vi "Overlay Feature Points-Sized.vi"(6 "Color":u32(colorbox)=16711680, 7 "Group":string, 8 "error in":errorcluster, 9 "Size":i32=5, 10 "Feature Points":cluster{"X":sgl, "Y":sgl}[](array[cluster]), 11 "Image":T1) -> (0 "error out":errorcluster, 3 "Image Out":T1)   [LabVIEW 2018]
doc: "Overlay targets at the location of the feature points in the specified colors."
uses:
  <vilib>/vision/Image Controls.llb/IMAQ Image.ctl
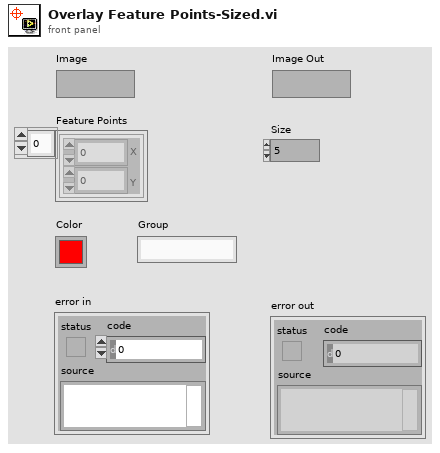
[diagram p1: front panel]
types:
  T1 = typedef "IMAQ Image.ctl" = refnum<image>
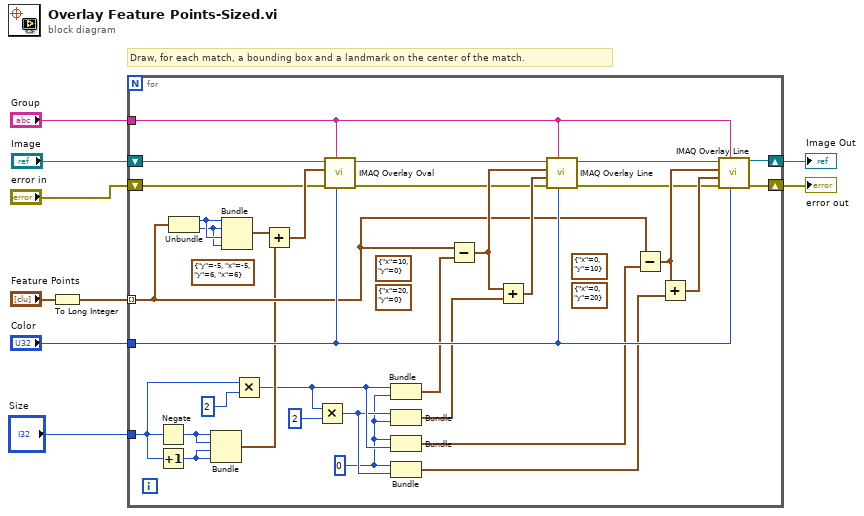
[diagram p0: block diagram]
diagram:
  # "Draw, for each match, a bounding box and a landmark on the center of the match."
  n1 = To Long Integer(number="Feature Points") -> (32bit integer=w6:cluster{"X":i32, "Y":i32}[])
  n2 = for {
    shift-right: [w39] -> w8
    shift-left: "Image" -> [w41]
    tunnel: w6 -> [w23] mode=indexing
    tunnel: "Color" -> [w40]
    tunnel: "Group" -> [w24]
    shift-right: [w25] -> w2
    shift-left: "error in" -> [w28]
    tunnel: "Size" -> [w19]
    w12 = 0 ("y")
    (unwired) cluster{"y":i32, "x":i32, "y":i32, "x":i32} {"y"=-5, "x"=-5, "y"=6, "x"=6} ("y")
    (unwired) cluster{"x":i32, "y":i32} {"x"=0, "y"=20} ("y")
    (unwired) cluster{"x":i32, "y":i32} {"x"=0, "y"=10} ("y")
    (unwired) cluster{"x":i32, "y":i32} {"x"=20, "y"=0} ("y")
    (unwired) cluster{"x":i32, "y":i32} {"x"=10, "y"=0} ("y")
    n3 = Negate(x=w19) -> (-x=w22:i32)
    n4 = Increment(x=w19) -> (x+1=w21:i32)
    n5 = Unbundle(w23) -> ("X"=w32:i32, "Y"=w31:i32)
    n6 = Bundle(w22, w22, w21, w21) -> (w20:cluster{i32, i32, i32, i32})  [unwired: 1 in]
    n7 = Bundle("X"=w32, "Y"=w31, "X"=w32, "Y"=w31) -> (w30:cluster{"X":i32, "Y":i32, "X":i32, "Y":i32})  [unwired: 1 in]
    n8 = Multiply(x=w19, y=2) -> (x*y=w14:i32)
    n9 = Add(x=w30, y=w20) -> (x+y=w29:cluster{i32, i32, i32, i32})
    n10 = Multiply(x=w14, y=2) -> (x*y=w13:i32)
    n11 = call "IMAQ Overlay Oval"("Color"=w40, "Group"=w24, "error in (no error)"=w28, "Bounding Rectangle"=w29, "Image"=w41) -> ("error out"=w27:errorcluster, "Image Out"=w33:T1)  [unwired: 5 in]
    n12 = Bundle(w14, "y"=w12) -> (w16:cluster{i32, "y":i32})  [unwired: 1 in]
    n13 = Bundle(w13, "y"=w12) -> (w15:cluster{i32, "y":i32})  [unwired: 1 in]
    n14 = Bundle("y"=w12, w14) -> (w11:cluster{"y":i32, i32})  [unwired: 1 in]
    n15 = Bundle("y"=w12, w13) -> (w10:cluster{"y":i32, i32})  [unwired: 1 in]
    n16 = Subtract(x=w23, y=w16) -> (x-y=w38:cluster{i32, i32})
    n17 = Add(x=w38, y=w15) -> (x+y=w37:cluster{i32, i32})
    n18 = call "IMAQ Overlay Line"("Color"=w40, "Group"=w24, "error in (no error)"=w27, "End Point"=w37, "Start Point"=w38, "Image"=w33) -> ("error out"=w26:errorcluster, "Image Out"=w34:T1)  [unwired: 4 in]
    n19 = Subtract(x=w23, y=w11) -> (x-y=w35:cluster{i32, i32})
    n20 = Add(x=w35, y=w10) -> (x+y=w36:cluster{i32, i32})
    n21 = call "IMAQ Overlay Line"("Color"=w40, "Group"=w24, "error in (no error)"=w26, "End Point"=w36, "Start Point"=w35, "Image"=w34) -> ("error out"=w25:errorcluster, "Image Out"=w39:T1)  [unwired: 4 in]
  }
  "Image Out" <- w8
  "error out" <- w2
